vi "SetLocalWaypoint.vi"(1 "Destination":T2={"Subsystem Id"=90, "Node Id"=1, "Component Id"=1}, 2 "Source":T2={"Subsystem Id"=3, "Node Id"=1, "Component Id"=1}, 3 "LocalWaypointRec":T1, 4 "PresenceVector":u8=2 format="%b") -> (0 "Encoded JAUS Message":string)   [LabVIEW 2009]
uses:
  Support Files/Address.ctl
  Support Files/LocalWaypointRec.ctl
panel:
  in  "Command Code":string="\u0004\u0003"
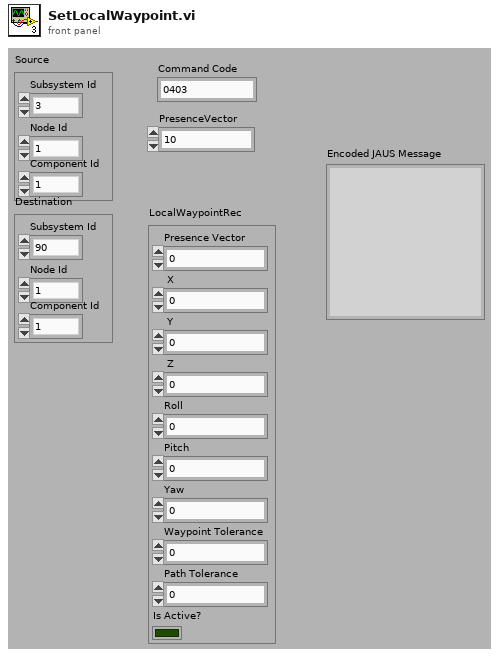
[diagram p1: front panel]
types:
  T1 = typedef "LocalWaypointRec.ctl" = cluster{"Presence Vector":u8, " X":dbl, " Y":dbl, " Z":dbl, "Roll":dbl, "Pitch":dbl, "Yaw":dbl, "Waypoint Tolerance":dbl, "Path Tolerance":dbl, "Is Active?":bool}
  T2 = typedef "Address.ctl" = cluster{"Subsystem Id":u16, "Node Id":u8, "Component Id":u8}
  T3 = cluster{"unsigned byte array[0]":u8, "unsigned byte array[1]":u8}
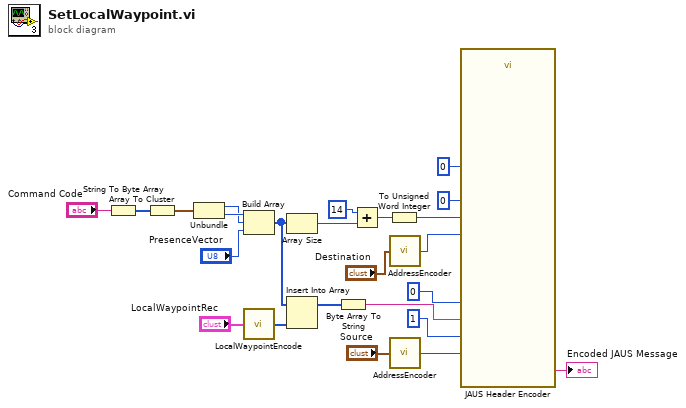
[diagram p0: block diagram]
diagram:
  n1 = String To Byte Array(string="Command Code") -> (unsigned byte array=w11:u8[])
  n2 = Array To Cluster(array=w11) -> (cluster=w12:T3)
  n3 = Unbundle(w12) -> ("unsigned byte array[0]"=w13:u8, "unsigned byte array[1]"=w14:u8)
  n4 = Build Array(w14, w13, "PresenceVector") -> (w1:u8[])
  n5 = call "LocalWaypointEncode.vi"("LocalWaypointRec"="LocalWaypointRec") -> ("Array"=w6:u8[])
  n6 = Array Size(array=w1) -> (size(s)=w8:i32)
  n7 = Insert Into Array(array=w1, new element=w6) -> (w5:u8[])  [unwired: 1 in]
  n8 = Byte Array To String(unsigned byte array=w5) -> (string=w2:string)
  n9 = Add(x=14, y=w8) -> (x+y=w15:i32)
  n10 = To Unsigned Word Integer(number=w15) -> (unsigned 16bit integer=w4:u16)
  n11 = call "AddressEncoder.vi"("Address Cluster"="Destination") -> ("Address"=w23:u32)
  n12 = call "AddressEncoder.vi"("Address Cluster"="Source") -> ("Address"=w24:u32)
  n13 = call "JAUS Header Encoder.vi"("Message Type (0-5)"=u8 0, "Data Size (8-23)"=w4, "Priority(40-41)"=u8 1, "Payload"=w2, "Source ID (80-95)"=w24, "Destination ID (48-79)"=w23, "Data Flags (46-47)"=u8 0, "Ack/Nak (44-45)"=u8 0) -> ("Encoded JAUS Message"=→"Encoded JAUS Message":string)  [unwired: 7 in]
